vi "PDC_GetExternalCount.vi"(8 "error in (no error)":errorcluster, 11 "DeviceNo":u32) -> (0 "error out":errorcluster, 1 "Out":u32, 2 "In":u32, 3 "ReturnValue":u32, 4 "ErrorCode":u32)   [LabVIEW 2015]
doc: "This VI retrieves the number of external input/output ports that the specified device has."
uses:
  PDCLIB.dll
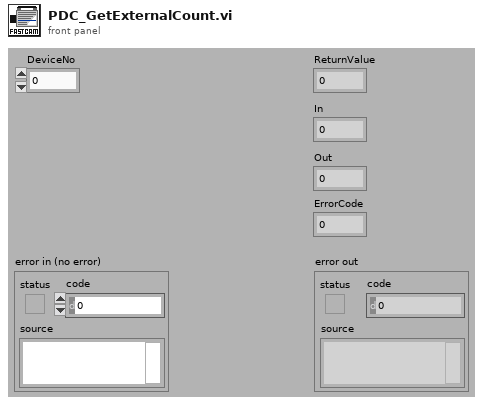
[diagram p1: front panel]
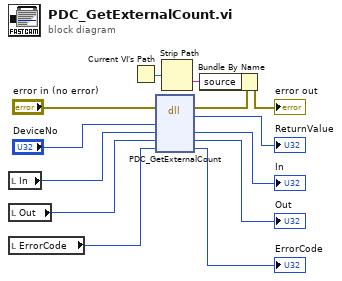
[diagram p0: block diagram]
diagram:
  n1 = local read "In"() -> (w7:u32)
  n2 = local read "Out"() -> (w6:u32)
  n3 = local read "ErrorCode"() -> (w10:u32)
  n4 = Current VI's Path() -> (path=w3:path)
  n5 = dll-call lib="PDCLIB.dll" fn="PDC_GetExternalCount"(error in="error in (no error)", "nDeviceNo"="DeviceNo", "pIn"=w7, "pOut"=w6, "pErrorCode"=w10) -> (error out=w2:errorcluster, "return type"=→"ReturnValue":u32, "pIn"=→"In":u32, "pOut"=→"Out":u32, "pErrorCode"=→"ErrorCode":u32)  [unwired: 3 in, 1 out]
  n6 = Strip Path(path=w3) -> (name=w4:string)  [unwired: 1 out]
  n7 = Bundle By Name(cluster=w2, "source"=w4) -> (→"error out":errorcluster)
